vi "Pockels Cal-Exctract cal data.vi"(9 "Processing Type (Interpolate)":T1, 11 "Pockels Cal table (full)":string[][](array[string])) -> (0 "OK":bool, 1 "Pockels Cal data (DBL)":dbl[][](array[numeric]), 2 "Index of last data row in the stripped cal data":i32, 3 "Pockels Cal data (strings)":string[][](array[string]))   [LabVIEW 2020]
uses:
  Typedefs/Pockels cal processing type.ctl
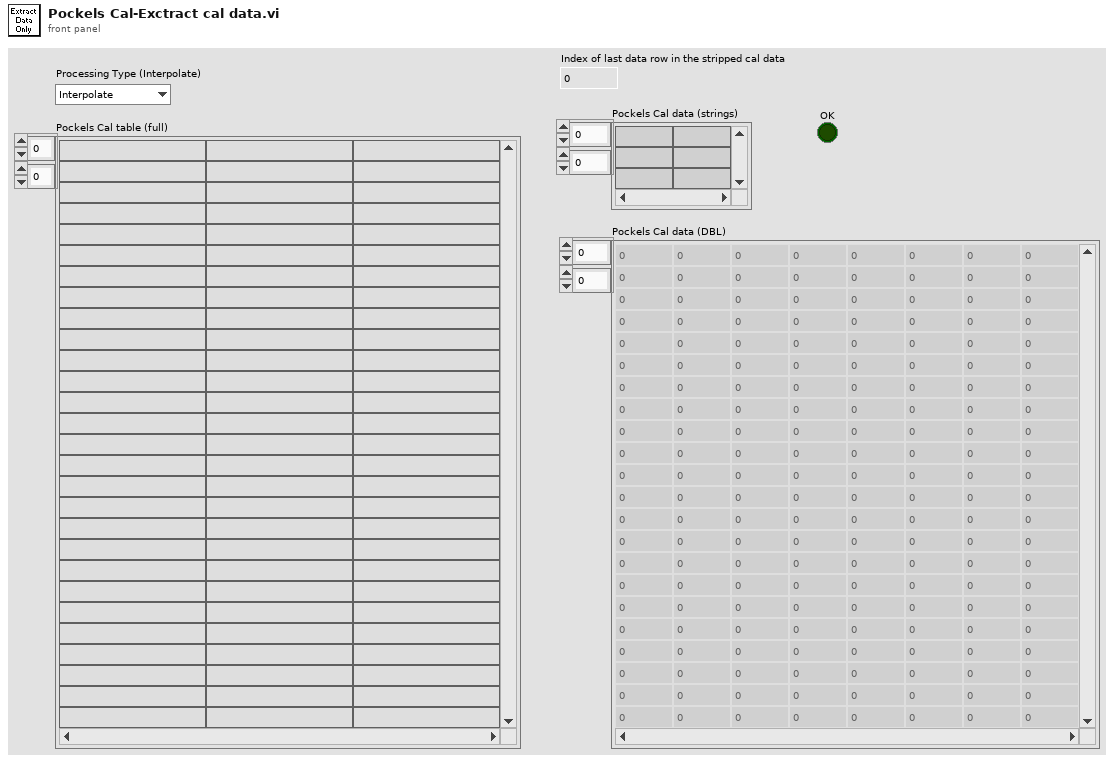
[diagram p1: front panel]
types:
  T1 = typedef "Pockels cal processing type.ctl" = enum16{"Interpolate", "Condense"}
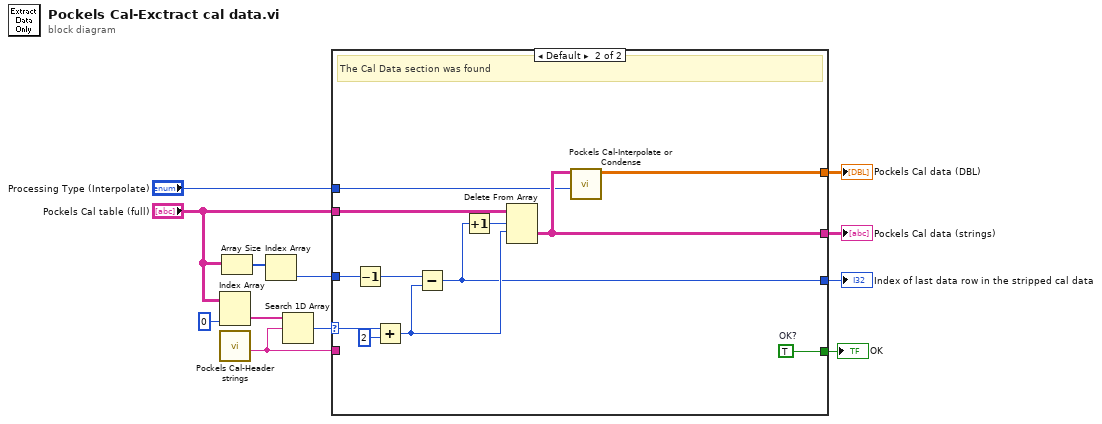
[diagram p0: block diagram]
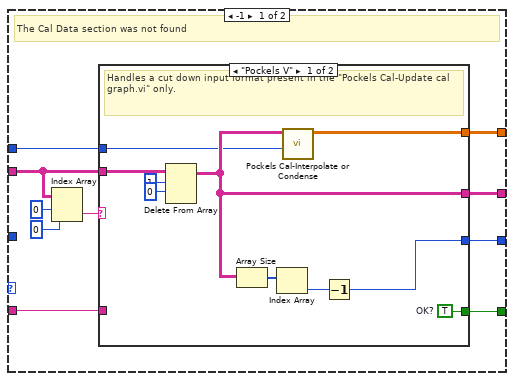
[diagram p2: hidden frame]
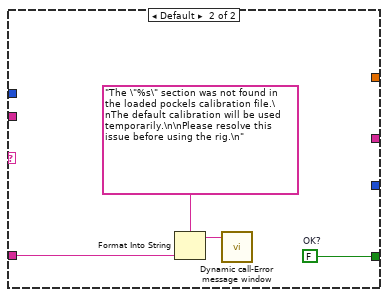
[diagram p3: hidden frame]
diagram:
  n1 = Index Array(array="Pockels Cal table (full)", index (col)=0 ("disabled index (col)")) -> (element=w7:string[])  [unwired: 1 in]
  n2 = call "Pockels Cal-Header strings.vi"() -> ("Cal data header string"=w3:string)  [unwired: 9 in, 2 out]
  n3 = Array Size(array="Pockels Cal table (full)") -> (size(s)=w11:i32[])
  n4 = Index Array(array=w11) -> (element=w12:i32)  [unwired: 1 in]
  n5 = Search 1D Array(1D array=w7, element=w3) -> (index of element=w4:i32)  [unwired: 1 in]
  n6 = case shown="Default" w4 {
    selector: w4 -> [_ w41]
    tunnel: w12 -> [_ w47]
    tunnel: "Pockels Cal table (full)" -> [w17 w46]
    tunnel: [w14 w43] -> w9
    tunnel: [w16 w38] -> w6
    tunnel: [w15 w39] -> w5
    tunnel: w3 -> [w22 _]
    tunnel: [w21 w40] -> w2
    tunnel: "Processing Type (Interpolate)" -> [w13 w37]
    frame -1 {
      # "The Cal Data section was not found"
      n7 = Index Array(array=w17, index (row)=0, index (col)=0 ("disabled index (col)")) -> (element=w18:string)
      n8 = case shown="\"Pockels V\"" w18 {
        tunnel: w22 -> [_ w34]
        tunnel: [w32 w33] -> w21
        tunnel: w17 -> [w31 _]
        tunnel: [w24 _] -> w16
        tunnel: [w25 _] -> w15
        tunnel: [w26 _] -> w14
        tunnel: w13 -> [w23 _]
        frame "Pockels V" {
          w32 = TRUE  # OK?
          # "Handles a cut down input format present in the \"Pockels Cal-Update cal graph.vi\" only."
          n9 = Delete From Array(array=w31, length=1, index (row)=0) -> (array with subset deleted=w25:string[][])  [unwired: 1 in, 1 out]
          n10 = Array Size(array=w25) -> (size(s)=w28:i32[])
          n11 = Index Array(array=w28) -> (element=w27:i32)  [unwired: 1 in]
          n12 = call "Pockels Cal-Interpolate or Condense.vi"("Processing Type (Interpolate)"=w23, "Pockels Cal table"=w25) -> ("Spline-Interpolated"=w24:dbl[][])  [unwired: 9 in]
          n13 = Decrement(x=w27) -> (x-1=w26:i32)
        }
        frame Default {
          w33 = FALSE  # OK?
          n14 = Format Into String(format string="The \"%s\" section was not found in the loaded pockels calibration file.\nThe default calibration will be used temporarily.\n\nPlease resolve this issue before using the rig.\n", w34) -> (resulting string=w35:string)  [unwired: 2 in, 1 out]
          n15 = call "Dynamic call-Error message window.vi"("Error Message"=w35) -> ()  [unwired: 10 in, 1 out]
        }
      }
    }
    frame Default {
      w40 = TRUE  # OK?
      # "The Cal Data section was found"
      n16 = Decrement(x=w47) -> (x-1=w48:i32)
      n17 = Add(x=w41, y=2) -> (x+y=w45:i32)
      n18 = Subtract(x=w48, y=w45) -> (x-y=w43:i32)
      n19 = Increment(x=w43) -> (x+1=w44:i32)
      n20 = Delete From Array "Delete From Array"(array=w46, length=w44, index (row)=w45) -> (deleted portion=w39:string[][])  [unwired: 1 in, 1 out]
      n21 = call "Pockels Cal-Interpolate or Condense.vi"("Processing Type (Interpolate)"=w37, "Pockels Cal table"=w39) -> ("Spline-Interpolated"=w38:dbl[][])  [unwired: 9 in]
    }
  }
  "Pockels Cal data (strings)" <- w5
  "Index of last data row in the stripped cal data" <- w9
  "Pockels Cal data (DBL)" <- w6
  "OK" <- w2
